vi "InsertItem.vi"(7 "Parent Tag":string, 8 "error in (no error)":errorcluster, 10 "MenuItem":refnum<class "MGI_MenuItem.lvclass">, 11 "MGI_VI in":refnum<class "MGI_VI.lvclass">) -> (0 "error out":errorcluster, 3 "MGI_VI out":refnum<class "MGI_VI.lvclass">)   [LabVIEW 2016, in "MGI_VI.lvclass"]
doc: "Authored by Derek E. Trepanier\nsupport@mooregoodideas.com\nwww.mooregoodideas.com\n\nCopyright (c) 2012, Moore Good Ideas, Inc.\n\nAll rights reserved.\n\nRedistribution and use in source and binary forms, with or without modification, are permitted provided that the following conditions are met:\n\n * Redistributions of source code must retain the above copyright notice, this list of conditions and the following disclaimer.\n * Redistributions in binary form must reproduce the above copyright notice, this list of conditions and the following disclaimer in the documentation and/or other materials provided with the distribution.\n * Neither the name of Moore Good Ideas, Inc. nor the names of its contributors may be used to endorse or promote products derived from this software without specific prior written permission.\n\nTHIS SOFTWARE IS PROVIDED BY THE COPYRIGHT HOLDERS AND CONTRIBUTORS \"AS IS\" AND ANY EXPRESS OR IMPLIED WARRANTIES, INCLUDING, BUT NOT LIMITED TO, THE IMPLIED WARRANTIES OF MERCHANTABILITY AND FITNESS FOR A PARTICULAR PURPOSE ARE DISCLAIMED. IN NO EVENT SHALL THE COPYRIGHT OWNER OR CONTRIBUTORS BE LIABLE FOR ANY DIRECT, INDIRECT, INCIDENTAL, SPECIAL, EXEMPLARY, OR CONSEQUENTIAL DAMAGES (INCLUDING, BUT NOT LIMITED TO, PROCUREMENT OF SUBSTITUTE GOODS OR SERVICES; LOSS OF USE, DATA, OR PROFITS; OR BUSINESS INTERRUPTION) HOWEVER CAUSED AND ON ANY THEORY OF LIABILITY, WHETHER IN CONTRACT, STRICT LIABILITY, OR TORT (INCLUDING NEGLIGENCE OR OTHERWISE) ARISING IN ANY WAY OUT OF THE USE OF THIS SOFTWARE, EVEN IF ADVISED OF THE POSSIBILITY OF SUCH DAMAGE."
uses:
  <userlib>/_MGI/Menu Building/MenuTypes/Vi/MGI_VI.lvclass
  <userlib>/_MGI/Menu Building/MenuItem/MGI_MenuItem.lvclass
  <userlib>/_MGI/Menu Building/MenuTypes/Vi/MGI_VI.lvclass/MGI_VI.ctl
  <userlib>/_MGI/Menu Building/MenuItem/Read Enabled.vi
  <userlib>/_MGI/Menu Building/MenuItem/Read Checked.vi
  <userlib>/_MGI/Menu Building/MenuItem/Read Full Tag.vi
  <userlib>/_MGI/Menu Building/MenuItem/Read Tag.vi
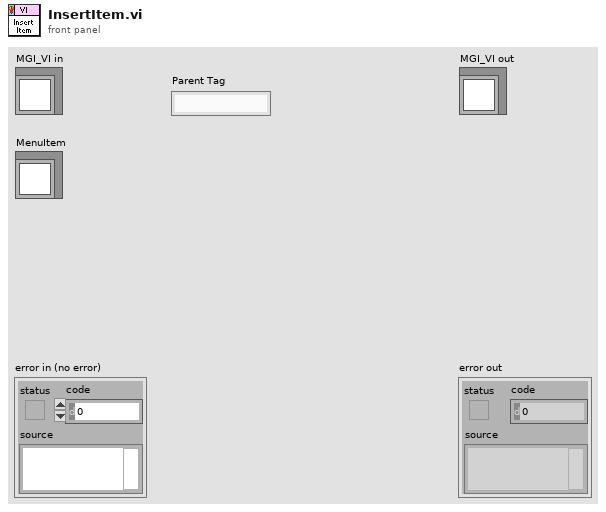
[diagram p1: front panel]
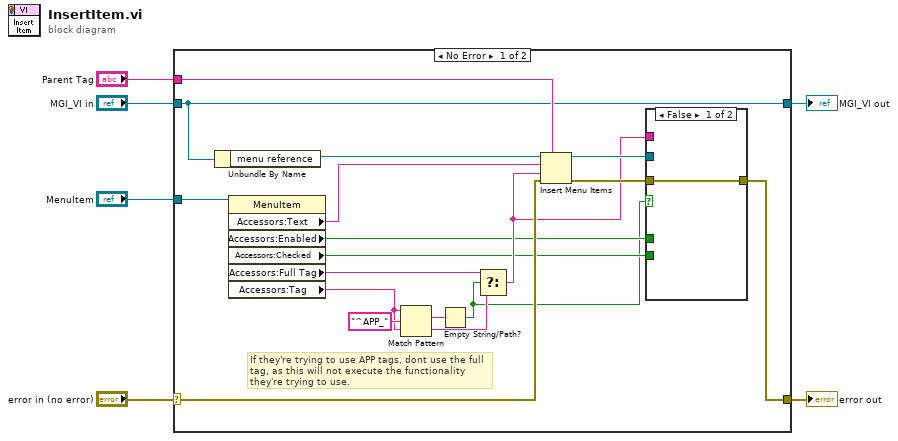
[diagram p0: block diagram]
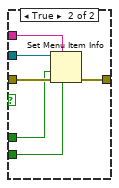
[diagram p2: hidden frame]
diagram:
  n1 = case shown="No Error" "error in (no error)" {
    selector: "error in (no error)" -> [w19 w32]
    tunnel: [w12 w32] -> w1
    tunnel: [w18 w31] -> w6
    tunnel: "MGI_VI in" -> [w18 w31]
    tunnel: "Parent Tag" -> [w22 _]
    tunnel: "MenuItem" -> [w21 _]
    frame No Error {
      # "If they're trying to use APP tags, dont use the full tag, as this will not execute the functionality they're trying to use."
      n2 = Unbundle By Name(w18) -> ("menu reference"=w23:refnum<k9>)
      n3 = property class="MenuItem"(reference=w21) -> ("Accessors:Text"=w20:string, "Accessors:Enabled"=w9:bool, "Accessors:Checked"=w8:bool, "Accessors:Full Tag"=w14:string, "Accessors:Tag"=w15:string)  [unwired: 1 in, 2 out]
      n4 = Match Pattern(string=w15, regular expression="^APP_") -> (match substring=w16:string)  [unwired: 1 in, 3 out]
      n5 = Empty String/Path?(string/path=w16) -> (empty?=w7:bool)
      n6 = Select(t=w14, s=w7, f=w15) -> (s? t:f=w10:string)
      n7 = Insert Menu Items(5:w22, 6:w19, 7:w10, 8:w20, 9:w23) -> (0:w13:errorcluster, 3:w11:refnum<k9>)  [unwired: 1 in, 1 out]
      n8 = case shown="False" w7 {
        tunnel: w13 -> [w24 w30]
        tunnel: [w24 w29] -> w12
        tunnel: w11 -> [_ w28]
        tunnel: w10 -> [_ w27]
        tunnel: w9 -> [_ w26]
        tunnel: w8 -> [_ w25]
        frame False {
        }
        frame True {
          n9 = Set Menu Item Info(6:w25, 7:w27, 8:w30, 9:w26, 11:w28) -> (0:w29:errorcluster)  [unwired: 2 in, 1 out]
        }
      }
    }
    frame Error {
    }
  }
  "error out" <- w1
  "MGI_VI out" <- w6
